vi "output power.vi"(7 "DAQ cluster in":T1 {"temp"."utility"."therm volt" format="%_6g"; "temp"."utility"."heat volt in" format="%_6g"; "temp"."utility"."heat volt out" format="%_6g"; "temp"."utility"."power out" format="%_6g"; "temp"."utility"."H Vmax" format="%_6g"; "temp"."T exec"."man power" format="%_6g"; "temp"."T exec"."exec setpoint" format="%_6g"; "temp"."T params"."Settle Time" step=1.0; "temp"."T params"."Settle Bandwidth" step=0.01; "temp"."T params"."Derivative Tme" step=0.01; "temp"."T params"."Integral Time" step=1.0; "temp"."T params"."Control Bandwidth" step=0.1; "temp"."T params"."Setpoint" step=0.1; "temp"."T status"."Setpoint" format="%_6g"; "temp"."T status"."Power" format="%_6g"; "temp"."T status"."Temp" format="%_6g"}, 11 "zero power":bool) -> (8 "DAQ cluster out":T1 {"temp"."utility"."therm volt" format="%_6g"; "temp"."utility"."heat volt in" format="%_6g"; "temp"."utility"."heat volt out" format="%_6g"; "temp"."utility"."power out" format="%_6g"; "temp"."utility"."H Vmax" format="%_6g"; "temp"."T exec"."man power" format="%_6g"; "temp"."T exec"."exec setpoint" format="%_6g"; "temp"."T params"."Settle Time" step=1.0; "temp"."T params"."Settle Bandwidth" step=0.01; "temp"."T params"."Derivative Tme" step=0.01; "temp"."T params"."Integral Time" step=1.0; "temp"."T params"."Control Bandwidth" step=0.1; "temp"."T params"."Setpoint" step=0.1; "temp"."T status"."Setpoint" format="%_6g"; "temp"."T status"."Power" format="%_6g"; "temp"."T status"."Temp" format="%_6g"}, 15 "error out":errorcluster)   [LabVIEW 2019]
doc: "This subVI is one of the states of the DAQ state machine in the bug experiment.\n\nThis state outputs the power to the heater.\n\nIt goes to the wait state next in pure temp contol mode, but goes to meas waveform next in the measure mode.\n\nIt has a zero power option for startup and close.\nPaul K Dixon\nP3600\nCSUSB Physics"
uses:
  typedefs/DAQ state cluster.ctl
  typedefs/DAQ state enum.ctl
  typedefs/temp cont cluster.ctl
  typedefs/temp exec cluster.ctl
  typedefs/temp mode enum.ctl
  typedefs/temp indicator.ctl
  typedefs/temp control status.ctl
  typedefs/PID control parameters.ctl
  typedefs/temp cont utility.ctl
  typedefs/measurement.ctl
  typedefs/wvfm acq params.ctl
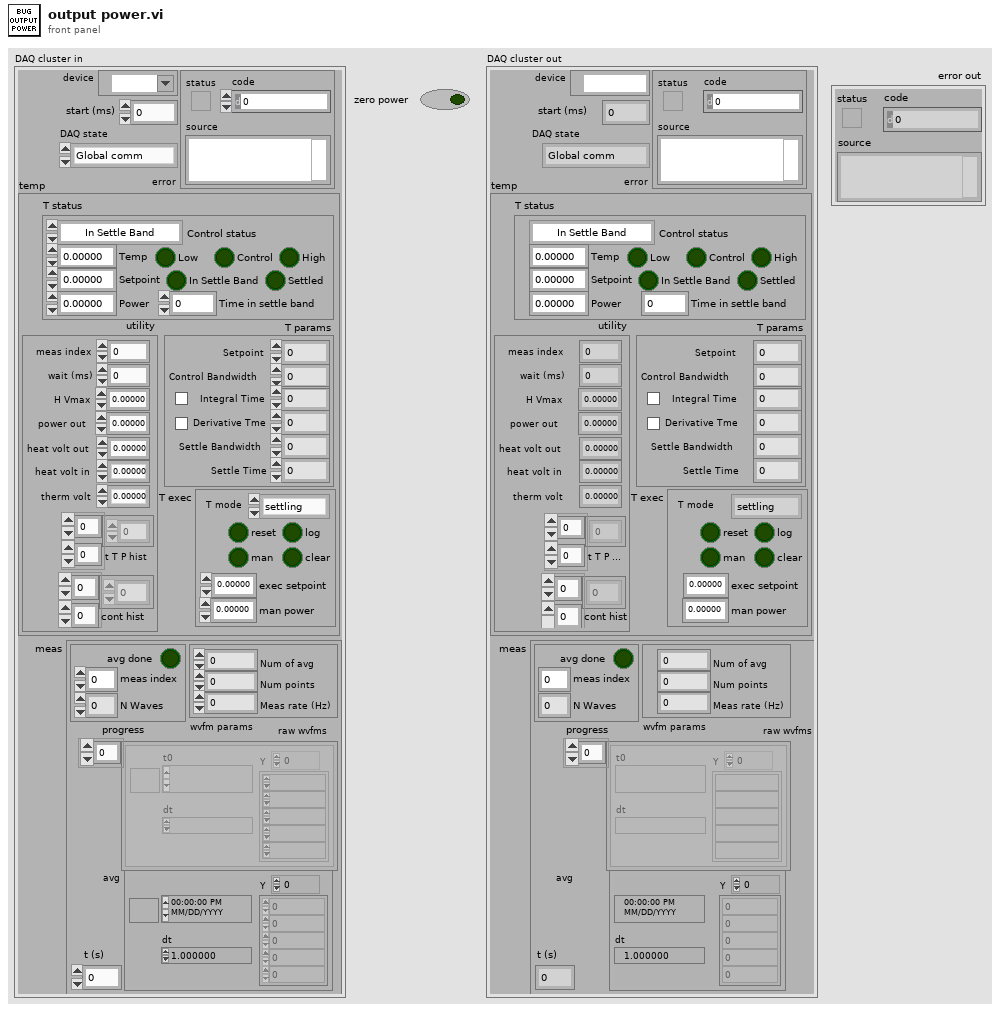
[diagram p1: front panel]
types:
  T1 = typedef "DAQ state cluster.ctl" = cluster{"DAQ state":T2, "temp":T3, "meas":T10, "device":tag, "error":errorcluster, "start (ms)":i32}
  T2 = typedef "DAQ state enum.ctl" = enum16{"Global comm", "Meas T & P", "PID power calc", "Man Power set", "Output Power", "Wait", "Meas wvfm", "Avg wvfm", "Exit"}
  T3 = typedef "temp cont cluster.ctl" = cluster{"T exec":T4, "T status":T6, "T params":T8, "utility":T9}
  T4 = typedef "temp exec cluster.ctl" = cluster{"T mode":T5, "exec setpoint":dbl, "reset":bool, "man power":dbl, "man":bool, "log":bool, "clear":bool}
  T5 = typedef "temp mode enum.ctl" = enum16{"settling", "measuring", "holding", "Exit"}
  T6 = typedef "temp indicator.ctl" = cluster{"Control status":T7, "Temp":dbl, "Power":dbl, "Time in settle band":dbl, "Settled":bool, "Low":bool, "High":bool, "Setpoint":dbl, "Control":bool, "In Settle Band":bool}
  T7 = typedef "temp control status.ctl" = enum16{"In Settle Band", "In Control Band", "Below Control Band", "Above Control Band"}
  T8 = typedef "PID control parameters.ctl" = cluster{"Setpoint":dbl, "Control Bandwidth":dbl, "Integral Time":dbl, "Int\nON":bool, "Derivative Tme":dbl, "Der\nON":bool, "Settle Bandwidth":dbl, "Settle Time":dbl}
  T9 = typedef "temp cont utility.ctl" = cluster{"meas index":i32, "wait (ms)":i32, "H Vmax":dbl, "power out":dbl, "heat volt out":dbl, "heat volt in":dbl, "therm volt":dbl, "t T P hist":dbl[][], "cont hist":dbl[][]}
  T10 = typedef "measurement.ctl" = cluster{"wvfm params":T11, "avg":waveform(dbl), "raw wvfms":waveform(dbl)[], "progress":cluster{"avg done":bool, "meas index":i32, "N waves":i32}, "t (s)":dbl}
  T11 = typedef "wvfm acq params.ctl" = cluster{"Num of avg":i32, "Num points":i32, "Meas rate (Hz)":dbl}
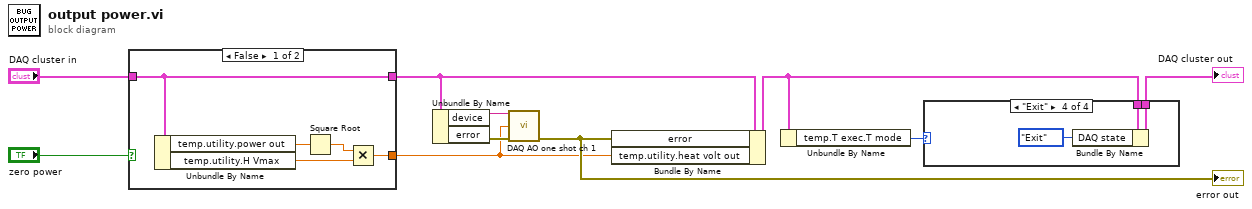
[diagram p0: block diagram]
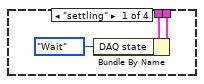
[diagram p2: hidden frame]
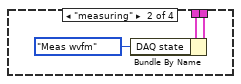
[diagram p3: hidden frame]
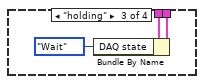
[diagram p4: hidden frame]
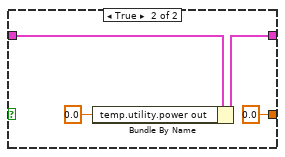
[diagram p5: hidden frame]
diagram:
  n1 = case shown="False" "zero power" {
    tunnel: "DAQ cluster in" -> [w11 w18]
    tunnel: [w12 0.0] -> w5
    tunnel: [w11 w17] -> w4
    frame False {
      n2 = Unbundle By Name(w11) -> ("temp.utility.power out"=w15:dbl, "temp.utility.H Vmax"=w13:dbl)
      n3 = Square Root(x=w15) -> (sqrt(x)=w14:dbl)
      n4 = Multiply(x=w14, y=w13) -> (x*y=w12:dbl)
    }
    frame True {
      n5 = Bundle By Name(cluster=w18, "temp.utility.power out"=0.0 ("T cont.utility.power out")) -> (w17:T1)
    }
  }
  n6 = Unbundle By Name(w4) -> ("device"=w9:tag, "error"=w8:errorcluster)
  n7 = call "DAQ AO one shot ch 1.vi"("device name"=w9, "Heater Voltage"=w5, "error in"=w8) -> ("error out"=w7:errorcluster)  [unwired: 11 in, 1 out]
  "error out" <- w7
  n8 = Bundle By Name(cluster=w4, "error"=w7, "temp.utility.heat volt out"=w5) -> (w2:T1)
  n9 = Unbundle By Name(w2) -> ("temp.T exec.T mode"=w1:T5)
  n10 = case shown="\"Exit\"" w1 {
    tunnel: [w22 w25 w28 w31] -> w10
    tunnel: w2 -> [w21 w24 w27 w30]
    frame "settling" {
      n11 = Bundle By Name(cluster=w21, "DAQ state"=DAQ_state_enum."Wait") -> (w22:T1)
    }
    frame "measuring" {
      n12 = Bundle By Name(cluster=w24, "DAQ state"=DAQ_state_enum."Meas wvfm") -> (w25:T1)
    }
    frame "holding" {
      n13 = Bundle By Name(cluster=w27, "DAQ state"=DAQ_state_enum."Wait") -> (w28:T1)
    }
    frame "Exit" {
      n14 = Bundle By Name(cluster=w30, "DAQ state"=DAQ_state_enum."Exit") -> (w31:T1)
    }
  }
  "DAQ cluster out" <- w10
